vi "readFanSpeed.vi"(8 "error in (no error)":errorcluster, 9 "id":T1=1, 10 "fanNumber":i32=1 min=1 max=4 step=1, 11 "CoolerControler in":refnum<class "CoolerControler.lvclass">) -> (0 "error out":errorcluster, 2 "fanSpeed":sgl, 3 "CoolerControler out":refnum<class "CoolerControler.lvclass">)   [LabVIEW 2016, in "CoolerControler.lvclass"]
uses:
  CoolerControler.lvclass
  typedefs/CoolerId.ctl
  SerialCommand/CoolerSerialCommand.lvclass
  typedefs/dataUnit.ctl
  typedefs/CoolerQuery.ctl
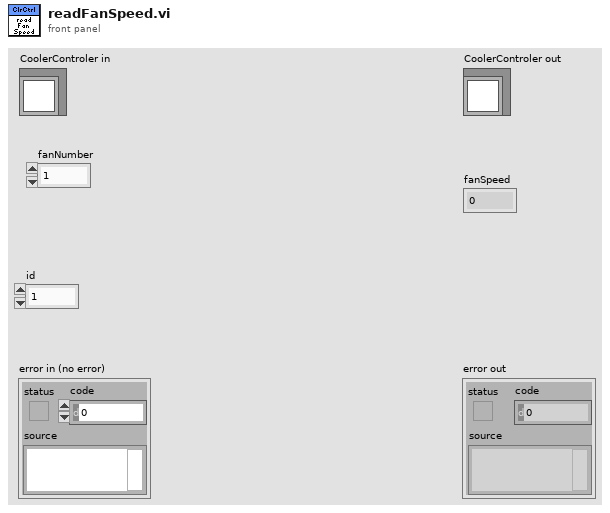
[diagram p1: front panel]
types:
  T1 = typedef "CoolerId.ctl" = u16
  T2 = typedef "dataUnit.ctl" = enum16{"temperature", "flow", "current", "PID", "fanSpeed", "time", "PWM", "TEDriveLevel", "Number"}
  T3 = typedef "CoolerQuery.ctl" = enum16{"ReadSerialWatchdog", "ReadControlSensor", "ReadSetTemperature", "ReadSupplyTemperature", "ReadExternalRTD", "ReadExternalThermistor", "ReadReturnTemperature", "ReadAmbientTemperature", "ReadProcessFlow", "ReadTECBank1Current", "ReadTECBank2Current", "ReadTEDriveLevel", "ReadAlarmStateLevel1", "ReadAlarmStateLevel21", "ReadAlarmStateLevel22", "ReadWarningStateLevel1", "ReadHighSupplyTempWarning", "ReadLowSupplyTempWarning", "ReadHighAmbientTempWarning", "ReadLowAmbientTempWarning", "ReadLowProcessFlowWarning", "ReadHighSupplyTempAlarm", "ReadLowSupplyTempAlarm", "ReadHighAmbientTempAlarm", "ReadLowAmbientTempAlarm", "ReadLowProcessFlowAlarm", "ReadPWMandRelayStatus", "ReadPIDStatus", "ReadUnitUpTime", "ReadFan1Speed", "ReadFan2Speed", "ReadFan3Speed", "ReadFan4Speed"}
  T4 = typedef "response.ctl" = cluster{"deviceId":string, "commandNumber":string, "errorActive":bool, "commandName":string, "responseData":string, "checkSum":string}
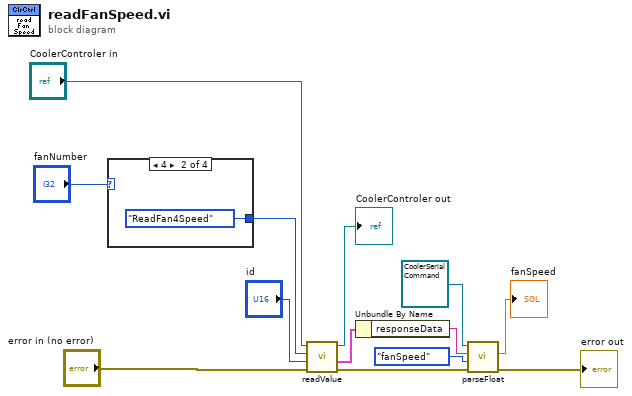
[diagram p0: block diagram]
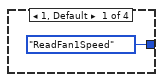
[diagram p2: hidden frame]
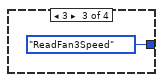
[diagram p3: hidden frame]
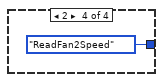
[diagram p4: hidden frame]
diagram:
  n1 = case shown="4" "fanNumber" {
    tunnel: [CoolerQuery."ReadFan1Speed" ("CoolerQuery") CoolerQuery."ReadFan4Speed" ("CoolerQuery") CoolerQuery."ReadFan3Speed" ("CoolerQuery") CoolerQuery."ReadFan2Speed" ("CoolerQuery")] -> w13
    frame 1, Default {
    }
    frame 4 {
    }
    frame 3 {
    }
    frame 2 {
    }
  }
  n2 = call "readValue.vi"("error in (no error)"="error in (no error)", "id"="id", "CoolerQuery"=w13, "CoolerControler in"="CoolerControler in") -> ("error out"=w9:errorcluster, "response out"=w11:T4, "CoolerControler out"=→"CoolerControler out":refnum<class "CoolerControler.lvclass">)  [unwired: 4 in, 1 out]
  n3 = Unbundle By Name(w11) -> ("responseData"=w10:string)
  n4 = call "parseFloat.vi"("error in (no error)"=w9, "unit"=dataUnit."fanSpeed", "commandData"=w10, "CoolerSerialCommand in"=refnum<class "CoolerSerialCommand.lvclass"> refnum) -> ("error out"=→"error out":errorcluster, "value"=→"fanSpeed":sgl)  [unwired: 4 in, 2 out]
